vi "dateiendung überprüfen.vi"(2 "filetype-array":string[](array[string]), 3 "Pfad":path) -> (0 "filename without extension":string, 1 "music file?":bool)   [LabVIEW 2010]
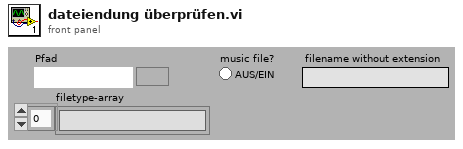
[diagram p1: front panel]
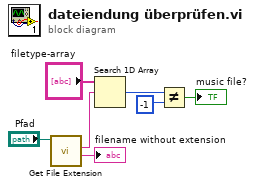
[diagram p0: block diagram]
diagram:
  n1 = call <vilib>:"Get File Extension.vi"("file"="Pfad") -> ("filename without extension"=→"filename without extension":string, "lowercase file extension"=w5:string)  [unwired: 1 in, 8 out]
  n2 = Search 1D Array(1D array="filetype-array", element=w5) -> (index of element=w4:i32)  [unwired: 1 in]
  n3 = Not Equal?(x=w4, y=-1) -> (x != y?=→"music file?":bool)
